vi "RIMAS Detector Read Scan Filenames.vi"(8 "Error In":errorcluster, 9 "Detector Config":T2={"Detector"=0, "Offsets"=[[0, 0, 0, 0, 0, 0, 0, 0, 0, 0, 0, 0, 0, 0, 0, 0, 0, 0, 0, 0, 0, 0, 0, 0, 0, 0, 0, 0, 0, 0, 0, 0]], "Detector Computer"={"Machine"="192.168.121.11", "Password"="", "FITS File Path"="", "Port"=44444, "Header Path"="", "Name"=""}, "FITS hdr template0"=path "", "FITS hdr template1"=path "", "FITS Data File Path"=path "", "FITS Detector Settings"={"Exp Time Short"=0.0, "# of Frames"=0.0, "Exp Time Long"=0.0, "# of Groups"=0.0, "Object Name"="", "Object"="", "Obs Type"="", "Image Type"="", "Observer"="", "Observer Affiliation"=""}, "Sim Folder"=path "", "Integration Mode"=enum."SSR", "Integration Time"=0.0, "Frame Int Time"=0.0} {"Offsets" format="%04x"; "Detector" items=["0", "1", "2"]}, 10 "Suffix data path":string, 11 "Detector Ref":refnum<k5>) -> (0 "Error Out":errorcluster, 1 "Image OK":bool, 2 "Image Data":T1 {"Detector #" items=["None", "YJ", "HK"]}, 3 "Detector Ref dup":refnum<k5>, 4 "Done":bool, 5 "Log":string)   [LabVIEW 2021]
uses:
  RIMAS Detector Config.ctl
  RIMAS Detector Server Config.ctl
  RIMAS Observation Config.ctl
  Detector enum Detector Integration Mode.ctl
  Detector Image typedef cluster.ctl
  <vilib>/regexp/Match Regular Expression.xnode
  Detector Class.lvclass
panel:
  out "Image":sgl[][](graph)
  out "FITS file acquired":path
  # "sec"
  # "sec"
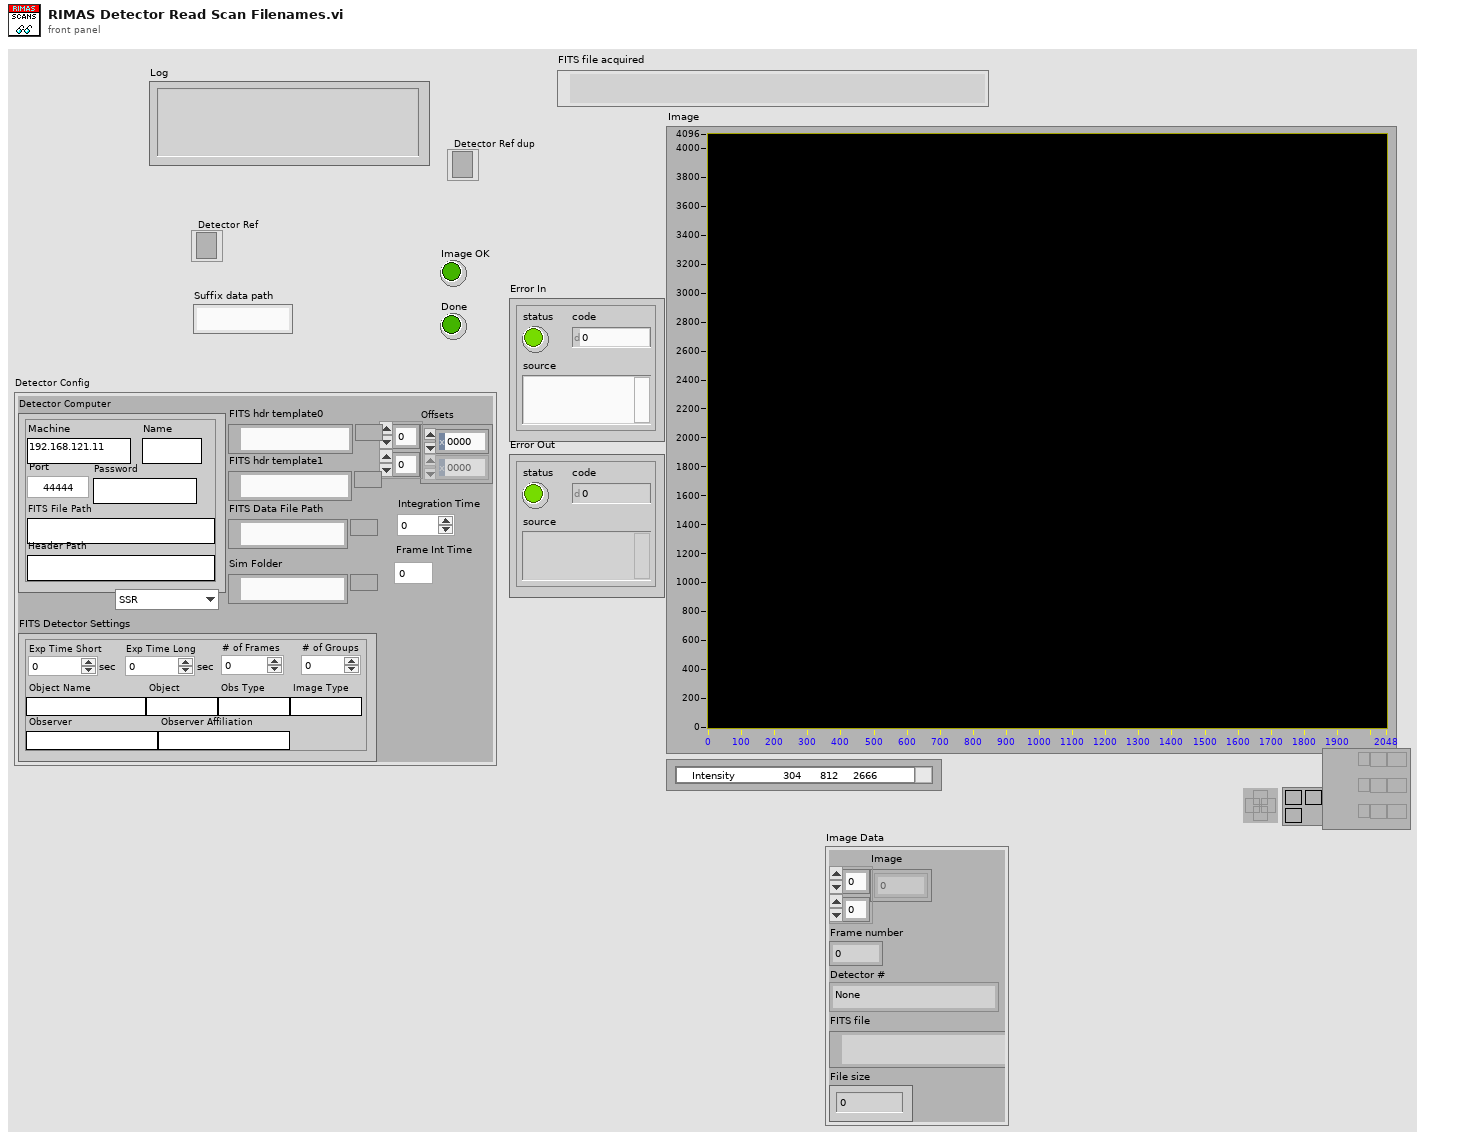
[diagram p1: front panel]
types:
  T1 = typedef "Detector Class.lvclass/Detector Image typedef cluster.ctl" = cluster{"Image":sgl[][], "Frame number":i32, "Detector #":u16, "FITS file":path, "File size":i64}
  T2 = typedef "RIMAS Detector Config.ctl" = cluster{"Detector":u16, "Offsets":u16[][], "Detector Computer":T3, "FITS hdr template0":path, "FITS hdr template1":path, "FITS Data File Path":path, "FITS Detector Settings":T4, "Sim Folder":path, "Integration Mode":T5, "Integration Time":dbl, "Frame Int Time":dbl}
  T3 = typedef "RIMAS Detector Server Config.ctl" = cluster{"Machine":string, "Password":string, "FITS File Path":string, "Port":u16, "Header Path":string, "Name":string}
  T4 = typedef "RIMAS Observation Config.ctl" = cluster{"Exp Time Short":dbl, "# of Frames":dbl, "Exp Time Long":dbl, "# of Groups":dbl, "Object Name":string, "Object":string, "Obs Type":string, "Image Type":string, "Observer":string, "Observer Affiliation":string}
  T5 = typedef "Detector enum Detector Integration Mode.ctl" = enum16{"SSR", "CDS", "MEAN", "MEDIAN", "MODE", "MIIN", "MAX"}
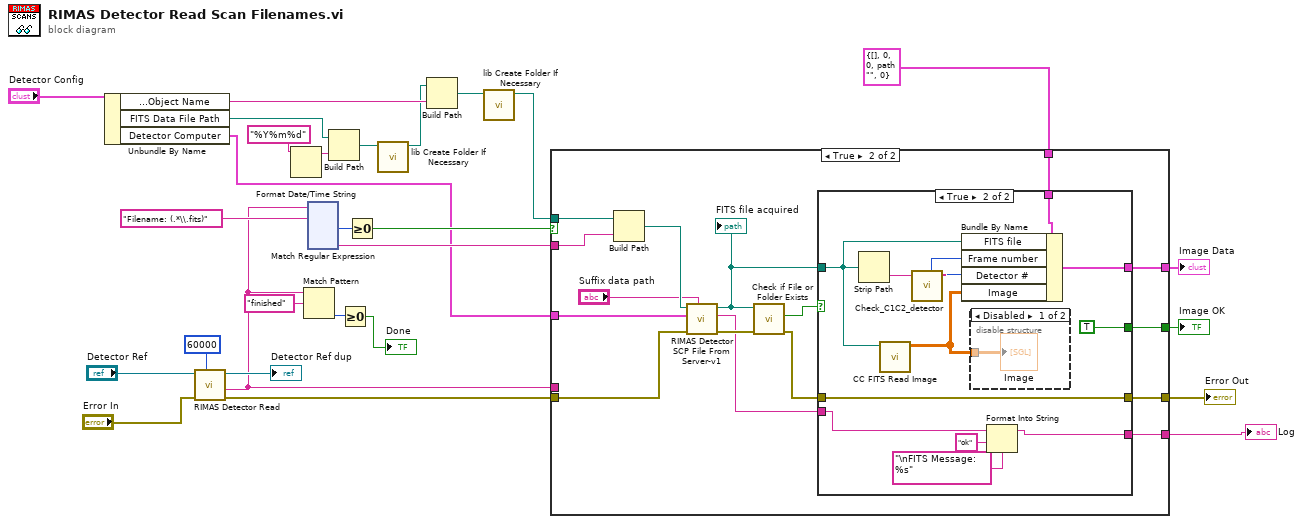
[diagram p0: block diagram]
diagram:
  n1 = Unbundle By Name("Detector Config") -> ("FITS Detector Settings.Object Name"=w6:string, "FITS Data File Path"=w7:path, "Detector Computer"=w5:T3)
  n2 = call "RIMAS Detector Read.vi"("timeout (ms)"=60000, "Error In"="Error In", "Detector Ref"="Detector Ref") -> ("Error Out"=w14:errorcluster, "First String"=w16:string, "Detector Ref dup"=→"Detector Ref dup":refnum<k5>)  [unwired: 5 in, 1 out]
  n3 = Format Date/Time String(time format string (%c)="%Y%m%d") -> (date/time string=w8:string)  [unwired: 2 in]
  n4 = Match Pattern(string=w16, regular expression="finished") -> (offset past match=w26:i32)  [unwired: 1 in, 3 out]
  n5 = xnode "Match Regular Expression"("input string"=w16, "regular expression"="Filename: (.*\\.fits)") -> ("offset past match"=w24:i32, "submatch 1"=w20:string)  [unwired: 4 in, 4 out]
  n6 = Build Path(base path=w7, name or relative path=w8) -> (appended path=w4:path)
  n7 = Greater Or Equal To 0?(x=w26) -> (x >= 0?=→"Done":bool)
  n8 = Greater Or Equal To 0?(x=w24) -> (x >= 0?=w21:bool)
  n9 = call "lib Create Folder If Necessary.vi"("Folder"=w4) -> ("Folder dup"=w3:path)  [unwired: 9 in, 1 out]
  n10 = Build Path(base path=w3, name or relative path=w6) -> (appended path=w2:path)
  n11 = call "lib Create Folder If Necessary.vi"("Folder"=w2) -> ("Folder dup"=w1:path)  [unwired: 9 in, 1 out]
  n12 = case shown="True" w21 {
    tunnel: w20 -> [_ w45]
    tunnel: w5 -> [_ w46]
    tunnel: w1 -> [_ w44]
    tunnel: w16 -> [w30 _]
    tunnel: [w30 w34] -> w15
    tunnel: w14 -> [w29 w38]
    tunnel: [w29 w35] -> w13
    tunnel: T1 {"Image"=[], "Frame number"=0, "Detector #"=0, "FITS file"=path "", "File size"=0} ("Image Data") -> [_ w33]
    tunnel: [_ w32] -> w11
    tunnel: [_ w31] -> w10
    frame False {
    }
    frame True {
      n13 = Build Path(base path=w44, name or relative path=w45) -> (appended path=w43:path)
      n14 = call "RIMAS Detector SCP File From Server-v1.vi"("Suffix data path"="Suffix data path", "Error In"=w38, "Detector Computer"=w46, "Local file path"=w43) -> ("Error Out"=w39:errorcluster, "log"=w37:string, "Dup Local file path"=w40:path)  [unwired: 5 in]
      "FITS file acquired" <- w40
      n15 = call <vilib>:"Check if File or Folder Exists.vi"("error in (no error)"=w39, "path"=w40) -> ("error out"=w36:errorcluster, "file or folder exists?"=w41:bool)  [unwired: 7 in, 1 out]
      n16 = case shown="True" w41 {
        tunnel: w40 -> [_ w51]
        tunnel: w37 -> [w47 w58]
        tunnel: w36 -> [w48 w60]
        tunnel: [w48 w60] -> w35
        tunnel: [w47 w57] -> w34
        tunnel: w33 -> [_ w56]
        tunnel: [_ w53] -> w32
        tunnel: [_ TRUE] -> w31
        frame False {
          # "report error"
        }
        frame True {
          n17 = Strip Path(path=w51) -> (name=w61:string)  [unwired: 1 out]
          n18 = call "CC FITS Read Image.vi"("FITS File Path"=w51) -> ("Image"=w50:sgl[][])  [unwired: 9 in, 1 out]
          n19 = call "Check_C1C2_detector.vi"("File name"=w61) -> ("Detector"=w54:u16, "Frame number"=w55:i32)  [unwired: 9 in]
          n20 = Bundle By Name(cluster=w56, "FITS file"=w51, "Frame number"=w55, "Detector #"=w54, "Image"=w50) -> (w53:T1)
          n21 = disable-structure shown="Disabled" {
            disable-tunnel: w50 -> [w62 _]
            frame Disabled {
              "Image" <- w62
            }
            frame Enabled {
            }
          }
          n22 = Format Into String(format string="\nFITS Message: %s", initial string=w58, "ok" ("input 1")) -> (resulting string=w57:string)  [unwired: 1 in, 1 out]
        }
      }
    }
  }
  "Error Out" <- w13
  "Log" <- w15
  "Image Data" <- w11
  "Image OK" <- w10
